vi "Exit.vi"(8 "error in (no error)":errorcluster, 11 "Old State":refnum<class "DC_Idle.lvclass">) -> (0 "error out":errorcluster, 3 "New State":refnum<class "DC_Idle.lvclass">)   [LabVIEW 2025, in "Display_Console.lvlib" / "DC_Idle.lvclass"]
doc: "This is an abstract method. Override this method to define the behavior when you leave the state."
uses:
  DC_Idle.lvclass
  DC_Idle.lvclass/DC_Idle.ctl
  Display_Console/Display_Console.lvclass
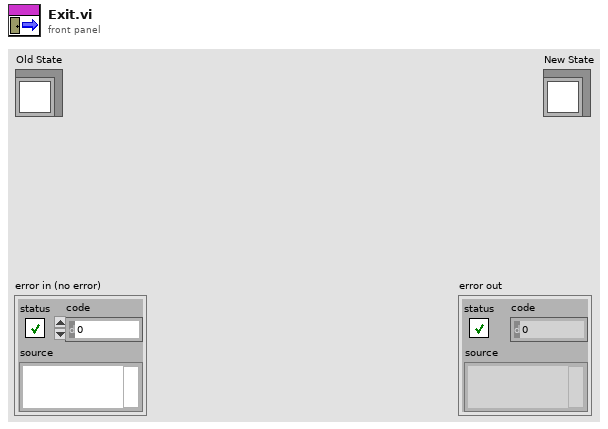
[diagram p1: front panel]
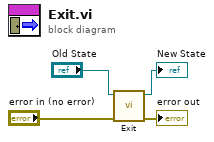
[diagram p0: block diagram]
diagram:
  n1 = call-parent "Exit.vi"("error in (no error)"="error in (no error)", "Old State"="Old State") -> ("error out"=→"error out":errorcluster, "New State"=→"New State":refnum<class "DC_Idle.lvclass">)  [unwired: 8 in]
